vi "input.vi"(8 "error in":errorcluster, 10 "input allocation":T1, 11 "System Diagnostics runtime in":refnum<class "System Diagnostics runtime.lvclass">) -> (0 "error out":errorcluster, 2 "input data":T1, 3 "System Diagnostics runtime out":refnum<class "System Diagnostics runtime.lvclass">)   [LabVIEW 2013, in "System Diagnostics runtime.lvclass"]
doc: "Provides an interface for reading data from a module at runtime. While this interface performs no operations, a child should provide an override which may read from any open sessions, references, or interfaces."
uses:
  System Diagnostics runtime.lvclass
  <vilib>/NI/Tag Bus/table/data table.ctl
  System Diagnostics runtime.lvclass/System Diagnostics runtime.ctl
  input user data.ctl
  <vilib>/Analysis/baseanly.llb/Mean (DBL).vi
  <resource>/objmgr/nisysapi.rc
  <vilib>/Analysis/NI_AALBase.lvlib
  <vilib>/NI/Tag Bus/table/data table.lvlib
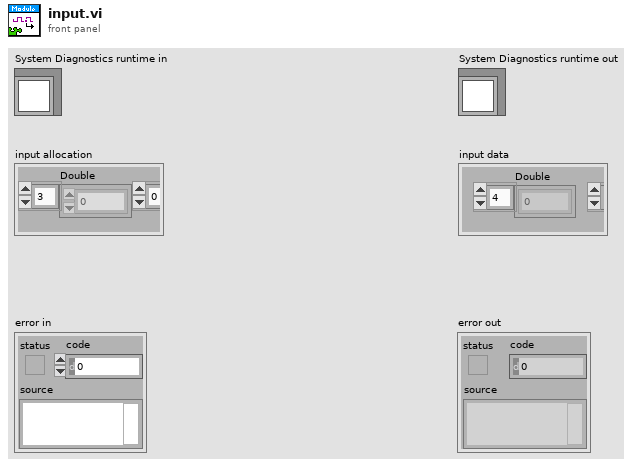
[diagram p1: front panel]
types:
  T1 = typedef "tag bus.lvlib/data table.lvlib/data table.ctl" = cluster{"Double":dbl[], "Single":sgl[], "I64":i64[], "I32":i32[], "I16":i16[], "I8":i8[], "U64":u64[], "U32":u32[], "U16":u16[], "U8":u8[], "Boolean":bool[], "String":string[], "Array of Double":cluster{"DBL Array":dbl[]}[], "Array of Single":cluster{"SGL Array":sgl[]}[], "Array of I64":cluster{"I64 Array":i64[]}[], "Array of I32":cluster{"I32 Array":i32[]}[], "Array of I16":cluster{"I16 Array":i16[]}[], "Array of I8":cluster{"I8 Array":i8[]}[], "Array of U64":cluster{"U64 Array":u64[]}[], "Array of U32":cluster{"U32 Array":u32[]}[], "Array of U16":cluster{"U16 Array":u16[]}[], "Array of U8":cluster{"U8 Array":u8[]}[], "Array of Boolean":cluster{"Boolean Array":bool[]}[], "Array of String":cluster{"String Array":string[]}[]}
  T2 = typedef "System Diagnostics runtime.lvclass/input user data.ctl" = cluster{"CPU load average":dbl, "timed structures load":dbl, "free memory":dbl, "contiguous memory":dbl}
  T3 = typedef "System Diagnostics configuration.lvclass/input data indices.ctl" = cluster{"Double.CPU load average":i32, "Double.timed structures load":i32, "Double.free memory":i32, "Double.contiguous memory":i32}
  T4 = typedef "NI_Real-Time Target Support.lvlib/RT CPU Load.ctl" = cluster{"Total (%)":dbl, "Time Critical (%)":dbl, "Timed Structures (%)":dbl, "High (%)":dbl, "Above Normal (%)":dbl, "Normal (%)":dbl, "Background (%)":dbl, "Idle (%)":dbl, "ISR (%)":dbl}
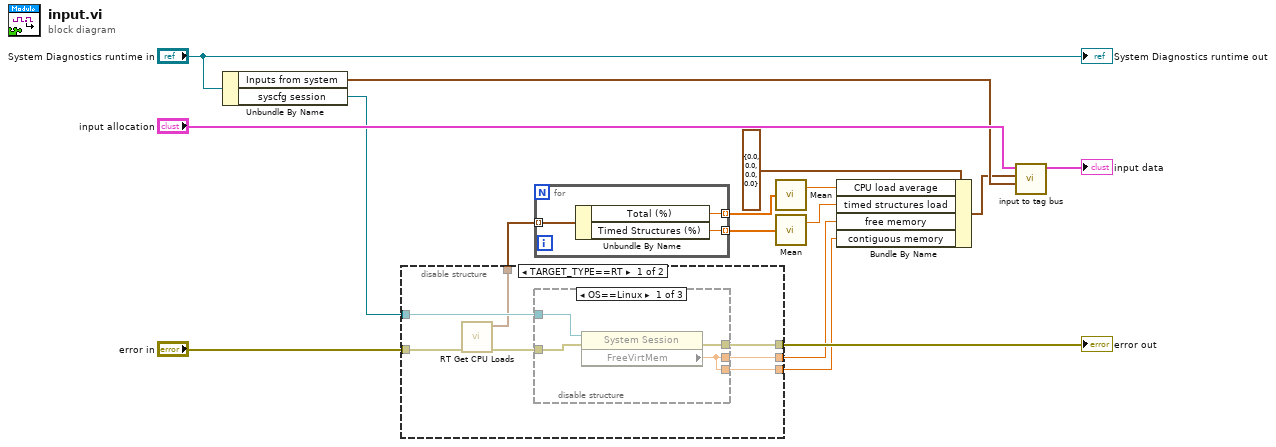
[diagram p0: block diagram]
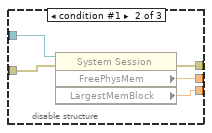
[diagram p2: hidden frame]
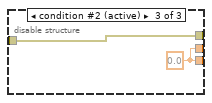
[diagram p3: hidden frame]
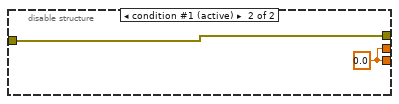
[diagram p4: hidden frame]
diagram:
  n1 = Unbundle By Name("System Diagnostics runtime in") -> ("Inputs from system"=w13:T3, "syscfg session"=w10:refnum<k21>)
  n2 = disable-structure shown="TARGET_TYPE==RT" {
    disable-tunnel: "error in" -> [w18 w36]
    disable-tunnel: w10 -> [w23 _]
    disable-tunnel: [w22 w36] -> w9
    disable-tunnel: [w21 w35] -> w4
    disable-tunnel: [w20 w35] -> w3
    disable-tunnel: [w19 _] -> w1
    frame condition #0 {
      n3 = call <vilib>:"RT Get CPU Loads.vi"("error in (no error)"=w18) -> ("error out"=w17:errorcluster, "CPU loads"=w19:T4[])  [unwired: 9 in]
      n4 = disable-structure shown="OS==Linux" {
        disable-tunnel: w17 -> [w27 w32 w33]
        disable-tunnel: w23 -> [w26 w31 _]
        disable-tunnel: [w25 w30 w33] -> w22
        disable-tunnel: [w24 w28 w34] -> w21
        disable-tunnel: [w24 w29 w34] -> w20
        frame condition #0 {
          n5 = property on="Property Node (System)" class="System Session"(reference=w26, error in=w27) -> (error out=w25:errorcluster, "FreeVirtMem"=w24:dbl)  [unwired: 1 out]
        }
        frame condition #1 {
          n6 = property on="Property Node (System)" class="System Session"(reference=w31, error in=w32) -> (error out=w30:errorcluster, "FreePhysMem"=w28:dbl, "LargestMemBlock"=w29:dbl)  [unwired: 1 out]
        }
        frame condition #2 (active) {
          w34 = 0.0
        }
      }
    }
    frame condition #1 (active) {
      w35 = 0.0
    }
  }
  "error out" <- w9
  n7 = for {
    tunnel: w1 -> [w39] mode=indexing
    tunnel: [w38] -> w8 mode=indexing
    tunnel: [w37] -> w7 mode=indexing
    n8 = Unbundle By Name(w39) -> ("Total (%)"=w38:dbl, "Timed Structures (%)"=w37:dbl)
  }
  n9 = call-poly <vilib>:"Mean.vi"("X"=w8) -> ("mean"=w5:dbl)  [unwired: 1 out]
  n10 = call-poly <vilib>:"Mean.vi"("X"=w7) -> ("mean"=w6:dbl)  [unwired: 1 out]
  n11 = Bundle By Name(cluster=T2 {"CPU load average"=0.0, "timed structures load"=0.0, "free memory"=0.0, "contiguous memory"=0.0} ("data cluster"), "CPU load average"=w5, "timed structures load"=w6, "free memory"=w4, "contiguous memory"=w3) -> (w11:T2)
  n12 = call "input to tag bus.vi"("indices"=w13, "data cluster"=w11, "tag bus in"="input allocation") -> ("tag bus out"=→"input data":T1)  [unwired: 8 in]
  "System Diagnostics runtime out" <- "System Diagnostics runtime in"
